vi "Configure SRQ.vi"(8 "error in (no error)":errorcluster, 10 "SRQ (F: OFF)":bool, 11 "VISA resource name":refnum<visa-resource-name>) -> (0 "error out":errorcluster, 3 "VISA resource name out":refnum<visa-resource-name>)   [LabVIEW 2021, in "Sorensen M9A Series.lvlib"]
doc: "This VI sets the Sorensen power supply's service request (SRQ) mode to either on or off. False == SRQ off, true == SRQ on. When on, an IEEE-488 GPIB service request will be generated for a variety of fault conditions. The power supply's default condition is SRQ OFF."
uses:
  Sorensen M9A Series.lvlib
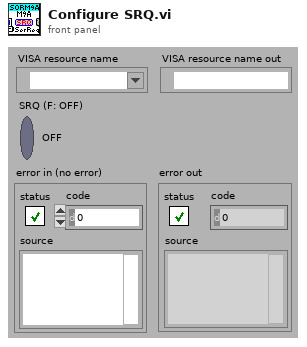
[diagram p1: front panel]
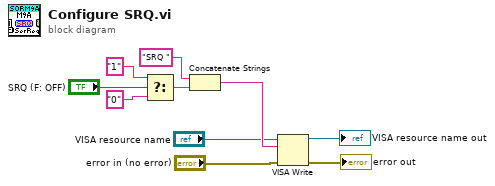
[diagram p0: block diagram]
diagram:
  n1 = Select(t="1", s="SRQ (F: OFF)", f="0") -> (s? t:f=w6:string)
  n2 = Concatenate Strings("SRQ ", w6) -> (w4:string)
  n3 = VISA Write(VISA resource name="VISA resource name", write buffer=w4, error in (no error)="error in (no error)") -> (VISA resource name out=→"VISA resource name out":refnum<visa-resource-name>, error out=→"error out":errorcluster)  [unwired: 1 out]
